vi "Untitled 1.vi"(11 "Characters to Write":string) -> (3 "Characters Read":string)   [LabVIEW 2017]
panel:
  out "Character Count":u32
  out "element":u8
  out "Characters Read 2":string
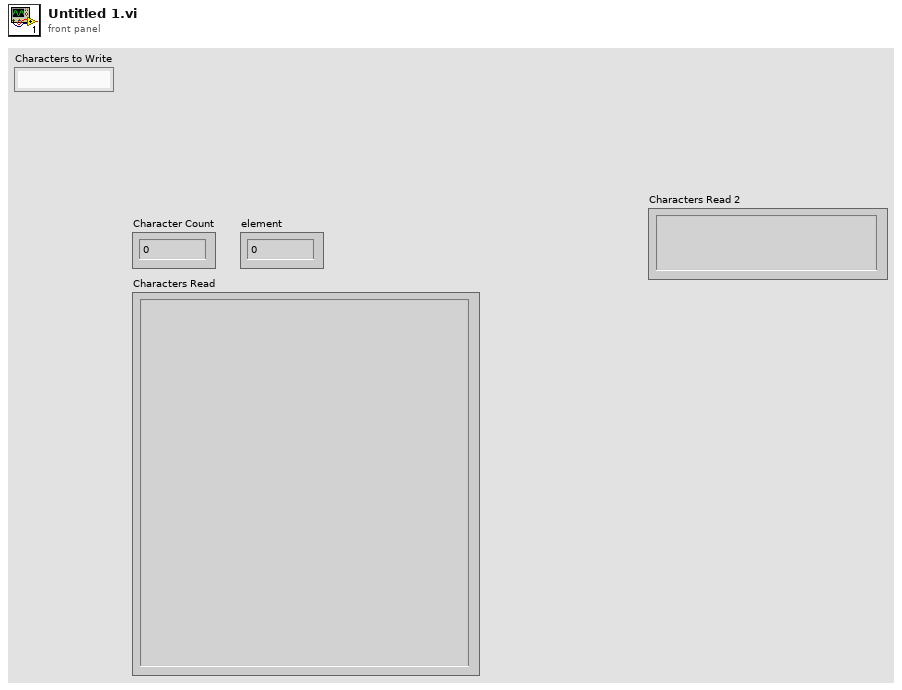
[diagram p1: front panel]
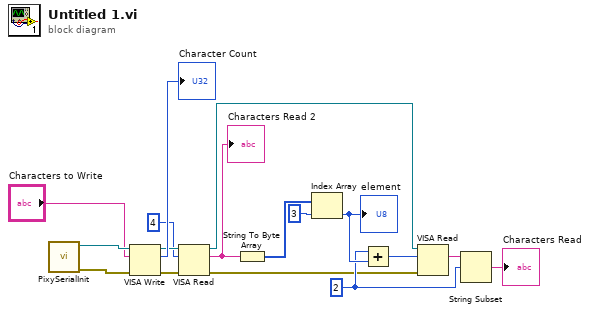
[diagram p0: block diagram]
diagram:
  w13 = u8 2 ("x")
  n1 = call "PixySerialInit.vi"() -> ("error out"=w10:errorcluster, "VISA resource name out"=w12:refnum<visa-resource-name>)  [unwired: 10 in]
  n2 = VISA Write(VISA resource name=w12, write buffer="Characters to Write", error in (no error)=w10) -> (VISA resource name out=w7:refnum<visa-resource-name>, return count=→"Character Count":u32, error out=w8:errorcluster)
  n3 = VISA Read(VISA resource name=w7, byte count=u32 4 ("Character Count"), error in (no error)=w8) -> (VISA resource name out=w2:refnum<visa-resource-name>, read buffer=w5:string, error out=w1:errorcluster)  [unwired: 1 out]
  "Characters Read 2" <- w5
  n4 = String To Byte Array(string=w5) -> (unsigned byte array=w15:u8[])
  n5 = Index Array(array=w15, index=3) -> (element=w17:u8)
  "element" <- w17
  n6 = Add(x=w13, y=w17) -> (x+y=w3:u8)
  n7 = VISA Read(VISA resource name=w2, byte count=w3, error in (no error)=w1) -> (read buffer=w4:string)  [unwired: 3 out]
  n8 = String Subset(string=w4, offset (0)=w13) -> (substring=→"Characters Read":string)  [unwired: 1 in]
